vi "AWG Start Pulses.vi"(8 "error in (no error)":errorcluster, 11 "awg session in":T1) -> (0 "error out":errorcluster, 3 "awg session out":T1)   [LabVIEW 2018, in "AWG.lvlib"]
doc: "AWG wrapper: Starts infinite pulse train with last set period."
uses:
  AWG.lvlib
  AWG Session.ctl
  AWG Type.ctl
  Agilent 33XXX Series/Agilent 33XXX Series.lvlib
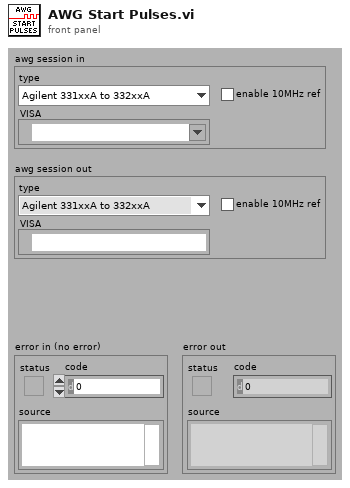
[diagram p1: front panel]
types:
  T1 = typedef "AWG.lvlib/AWG Session.ctl" = cluster{"type":T2, "VISA":refnum<visa-resource-name>, "enable 10MHz ref":bool}
  T2 = typedef "AWG.lvlib/AWG Type.ctl" = enum16{"Agilent 331xxA to 332xxA", "Agilent 335xxA to 336xxA", "Tektronix AFG3101C", "dummy"}
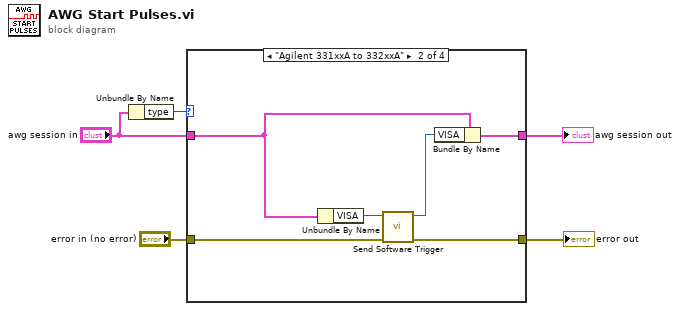
[diagram p0: block diagram]
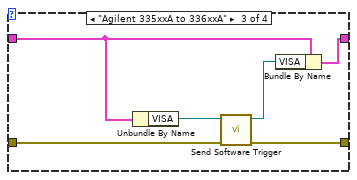
[diagram p3: hidden frame]
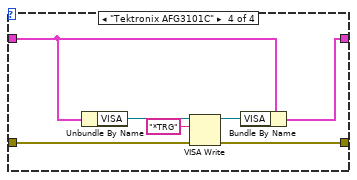
[diagram p4: hidden frame]
diagram:
  n1 = Unbundle By Name("awg session in") -> ("type"=w5:T2)
  n2 = case shown="\"Agilent 331xxA to 332xxA\"" w5 {
    tunnel: "error in (no error)" -> [w7 w8 w14 w21]
    tunnel: [w7 w11 w16 w26] -> w3
    tunnel: "awg session in" -> [w6 w12 w19 w25]
    tunnel: [w6 w13 w18 w22] -> w1
    frame Default {
    }
    frame "Agilent 331xxA to 332xxA" {
      n3 = Unbundle By Name(w12) -> ("VISA"=w9:refnum<visa-resource-name>)
      n4 = call "Send Software Trigger.vi"("error in (no error)"=w8, "VISA resource name"=w9) -> ("error out"=w11:errorcluster, "VISA resource name out"=w10:refnum<visa-resource-name>)  [unwired: 8 in]
      n5 = Bundle By Name(cluster=w12, "VISA"=w10) -> (w13:T1)
    }
    frame "Agilent 335xxA to 336xxA" {
      n6 = Unbundle By Name(w19) -> ("VISA"=w15:refnum<visa-resource-name>)
      n7 = call "Send Software Trigger.vi"("error in (no error)"=w14, "VISA resource name"=w15) -> ("error out"=w16:errorcluster, "VISA resource name out"=w17:refnum<visa-resource-name>)  [unwired: 8 in]
      n8 = Bundle By Name(cluster=w19, "VISA"=w17) -> (w18:T1)
    }
    frame "Tektronix AFG3101C" {
      n9 = Unbundle By Name(w25) -> ("VISA"=w20:refnum<visa-resource-name>)
      n10 = VISA Write(VISA resource name=w20, write buffer="*TRG", error in (no error)=w21) -> (VISA resource name out=w24:refnum<visa-resource-name>, error out=w26:errorcluster)  [unwired: 1 out]
      n11 = Bundle By Name(cluster=w25, "VISA"=w24) -> (w22:T1)
    }
  }
  "error out" <- w3
  "awg session out" <- w1
